vi "Get Application Manager.vi"(8 "Error In":errorcluster, 11 "Engine In":refnum<k7>) -> (0 "Error Out":errorcluster, 2 "Application Manager":refnum<k7>, 3 "Engine Out":refnum<k7>)   [LabVIEW 2021, in "Seq Edit Quick Drop.lvlib"]
uses:
  Seq Edit Quick Drop.lvlib
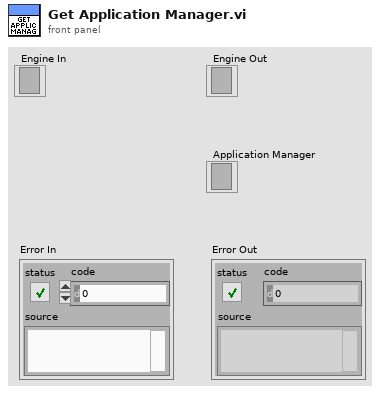
[diagram p1: front panel]
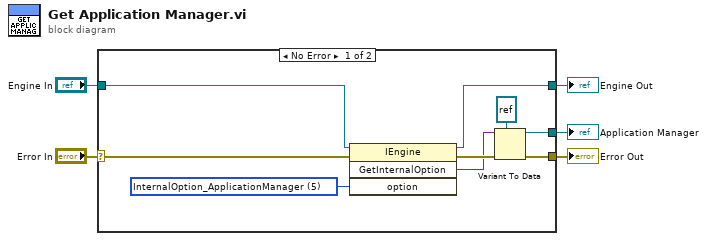
[diagram p0: block diagram]
diagram:
  n1 = case shown="No Error" "Error In" {
    selector: "Error In" -> [w6 w16]
    tunnel: [w13 _] -> w5
    tunnel: [w12 w15] -> w4
    tunnel: "Engine In" -> [w11 w15]
    tunnel: [w7 w16] -> w2
    frame No Error {
      w8 = 5 items=["InternalOption_WarnOnAPICallThroughDispatchInterface"=1, "InternalOption_AutomationAdapterUsesDispatchForDualInterfaces"=2, "InternalOption_UpdateExternalEnvironments"=3, "InternalOption_ApplicationManager"=5, "InternalOption_DisableFloatingWindowsForModalDialogs"=10] ("option")
      n2 = invoke class="IEngine" method="GetInternalOption"(reference=w11, error in=w6, "option"=w8) -> (reference out=w12:refnum<k7>, error out=w14:errorcluster, "GetInternalOption"=w9:variant)  [unwired: 1 in, 1 out]
      n3 = Variant To Data(error in=w14, type=refnum<k7> refnum ("ApplicationMgr"), Variant=w9) -> (data=w13:refnum<k7>, error out=w7:errorcluster)
    }
    frame Error {
    }
  }
  "Application Manager" <- w5
  "Engine Out" <- w4
  "Error Out" <- w2
